vi "findIndices4MissingData (SubVI).vi"(1 "data":dbl[](array[numeric])) -> (0 "missing data indices":i32[][](array[numeric]))   [LabVIEW 2017]
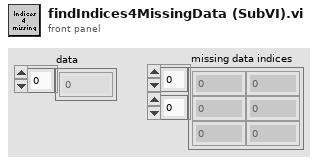
[diagram p1: front panel]
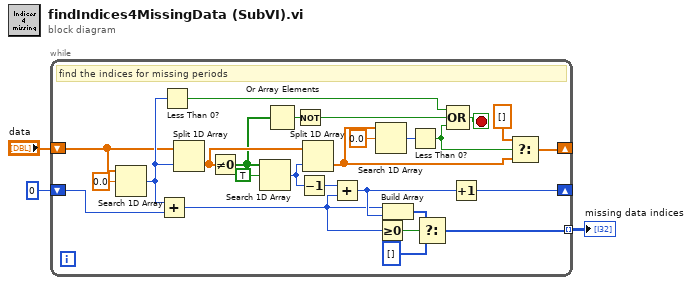
[diagram p0: block diagram]
diagram:
  n1 = while {
    shift-right: [w20] -> _
    shift-left: "data" -> [w11]
    shift-right: [w12] -> _
    shift-left: 0 ("index of element") -> [w26]
    tunnel: [w5] -> w2 mode=indexing
    stop <- w18 stop-if-true
    # "find the indices for missing periods"
    n2 = Search 1D Array(1D array=w11, element=0.0) -> (index of element=w17:i32)  [unwired: 1 in]
    n3 = Add(x=w17, y=w26) -> (x+y=w4:i32)
    n4 = Less Than 0?(x=w17) -> (x < 0?=w10:bool)
    n5 = Split 1D Array(array=w11, index=w17) -> (second subarray=w8:dbl[])  [unwired: 1 out]
    n6 = Not Equal To 0?(x=w8) -> (x != 0?=w7:bool[])
    n7 = Search 1D Array(1D array=w7, element=TRUE) -> (index of element=w27:i32)  [unwired: 1 in]
    n8 = Or Array Elements(Boolean array=w7) -> (logical OR=w9:bool)
    n9 = Not(x=w9) -> (.not. x?=w6:bool)
    n10 = Decrement(x=w27) -> (x-1=w25:i32)
    n11 = Split 1D Array(array=w8, index=w27) -> (second subarray=w22:dbl[])  [unwired: 1 out]
    n12 = Add(x=w25, y=w4) -> (x+y=w13:i32)
    n13 = Search 1D Array(1D array=w22, element=0.0) -> (index of element=w23:i32)  [unwired: 1 in]
    n14 = Greater Or Equal To 0?(x=w4) -> (x >= 0?=w15:bool)
    n15 = Build Array(w4, w13) -> (w16:i32[])
    n16 = Less Than 0?(x=w23) -> (x < 0?=w19:bool)
    n17 = Select(t=w16, s=w15, f=i32[] []) -> (s? t:f=w5:i32[])
    n18 = Compound Arithmetic op=OR(w10, w6, w19) -> (w18:bool)
    n19 = Increment(x=w13) -> (x+1=w12:i32)
    n20 = Select(t=dbl[] [], s=w19, f=w22) -> (s? t:f=w20:dbl[])
  }
  "missing data indices" <- w2
